vi "Indicator Color Selector.vi"(9 "Comparitor":dbl[](array[numeric]), 11 "Input Array":dbl[](array[numeric])) -> (1 "Color Array":u32[](array[numeric]), 3 "Output Array":dbl[](array[numeric]))   [LabVIEW 2013]
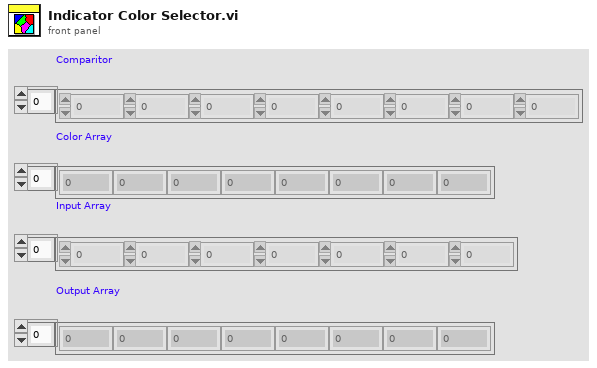
[diagram p1: front panel]
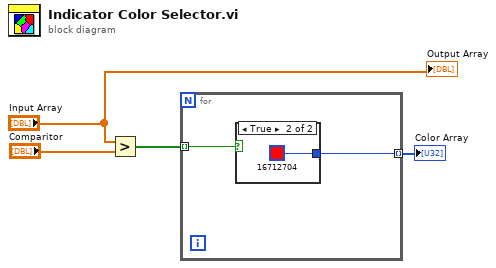
[diagram p0: block diagram]
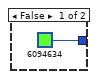
[diagram p2: hidden frame]
diagram:
  n1 = Greater?(x="Input Array", y="Comparitor") -> (0:w3:bool[])
  n2 = for {
    tunnel: w3 -> [w6] mode=indexing
    tunnel: [w5] -> w2 mode=indexing
    n3 = case shown="True" w6 {
      tunnel: [u32 6094634 u32 16712704] -> w5
      frame False {
      }
      frame True {
      }
    }
  }
  "Color Array" <- w2
  "Output Array" <- "Input Array"
